vi "Stop Core.vi"(10 "final error code":i32, 11 "client in":refnum<class "client.lvclass">) -> (3 "client out":refnum<class "client.lvclass">)   [LabVIEW 2016, in "client.lvlib" / "client.lvclass"]
doc: "(<B>Filename</B>: Actor Framework.lvlib:Actor.lvclass:Stop Core.vi)\n\nDefines what the actor does before it stops. Use the <B>final error code</B> input to determine whether the actor shut down in response to an error.\n\nBy default, this method does nothing. A descendant class may override it to define behavior, such as shutting down any processes the actor initiated in its override of the Actor Core method."
uses:
  client.lvclass
  client.lvclass/client.ctl
  <vilib>/ActorFramework/Actor/Actor.lvclass
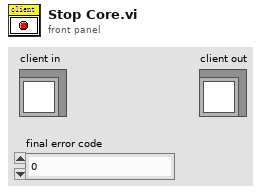
[diagram p1: front panel]
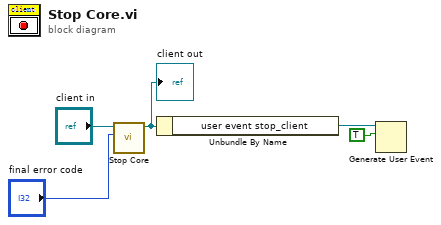
[diagram p0: block diagram]
diagram:
  n1 = call-parent "Stop Core.vi"("final error code"="final error code", "Actor in"="client in") -> ("Actor out"=w2:refnum<class "client.lvclass">)  [unwired: 9 in]
  "client out" <- w2
  n2 = Unbundle By Name(w2) -> ("user event stop_client"=w3:refnum<user-event>)
  n3 = Generate User Event(user event=w3, event data cluster=TRUE) -> ()  [unwired: 2 in, 2 out]
